vi "E4440A_PSA_Configure_Marker.vi"(0 "VISA resource name":refnum<visa-resource-name>, 1 "X (0 Hz)":dbl, 2 "Center X (0)":dbl, 3 "X Span (0)":dbl, 5 "Active Marker (1: Marker1)":u16(ring)=1 items=["Marker1"=1, "Marker2"=2, "Marker3"=3, "Marker4"=4], 7 "Marker Type (1: Position)":u16(ring)=1 items=["Off", "Position", "Delta", "Band", "Span Pair"], 9 "Readout (0: Frequency)":u16(ring) items=["Frequency", "Time", "Inverse Time", "Period"], 11 "error in (no error)":errorcluster, 12 "X Start (0)":dbl, 13 "X Stop (0)":dbl) -> (4 "VISA resource name out":refnum<visa-resource-name>, 15 "error out":errorcluster)   [LabVIEW 2015]
doc: "Configures the marker type settings of the selected marker."
panel:
  # "Span Pair"
  # "Band"
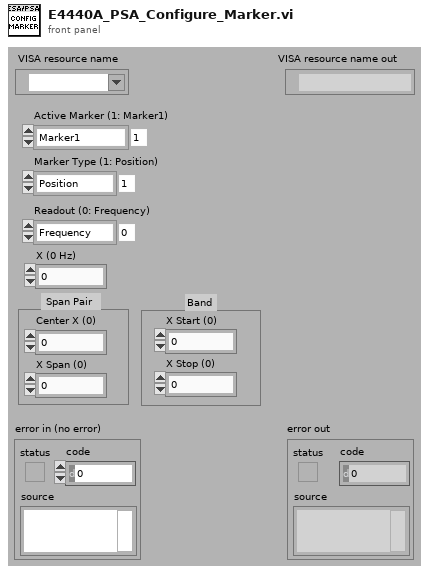
[diagram p1: front panel]
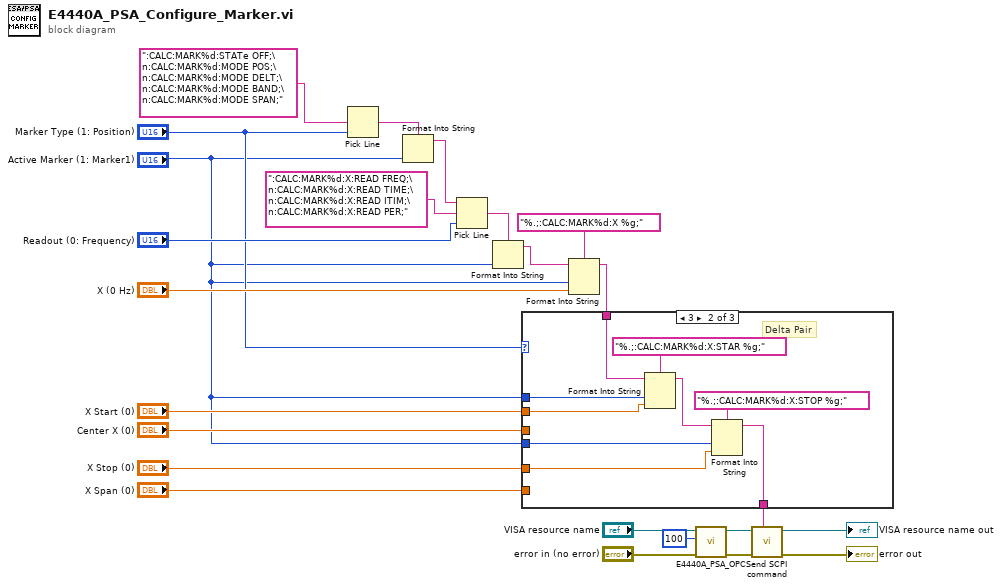
[diagram p0: block diagram]
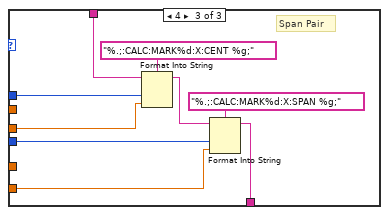
[diagram p3: hidden frame]
diagram:
  n1 = Pick Line(multi-line string=":CALC:MARK%d:STATe OFF;\n:CALC:MARK%d:MODE POS;\n:CALC:MARK%d:MODE DELT;\n:CALC:MARK%d:MODE BAND;\n:CALC:MARK%d:MODE SPAN;", line index="Marker Type (1: Position)") -> (output string=w22:string)  [unwired: 1 in]
  n2 = Format Into String(format string=w22, "Active Marker (1: Marker1)") -> (resulting string=w19:string)  [unwired: 2 in, 1 out]
  n3 = Pick Line(string ("")=w19, multi-line string=":CALC:MARK%d:X:READ FREQ;\n:CALC:MARK%d:X:READ TIME;\n:CALC:MARK%d:X:READ ITIM;\n:CALC:MARK%d:X:READ PER;", line index="Readout (0: Frequency)") -> (output string=w18:string)
  n4 = Format Into String(format string=w18, "Active Marker (1: Marker1)") -> (resulting string=w16:string)  [unwired: 2 in, 1 out]
  n5 = Format Into String(format string="%.;:CALC:MARK%d:X %g;", initial string=w16, "Active Marker (1: Marker1)", "X (0 Hz)") -> (resulting string=w13:string)  [unwired: 1 in, 1 out]
  n6 = case shown="3" "Marker Type (1: Position)" {
    tunnel: "Active Marker (1: Marker1)" -> [_ w31 w39]
    tunnel: "Active Marker (1: Marker1)" -> [_ w30 w38]
    tunnel: w13 -> [w25 w29 w40]
    tunnel: [w25 w28 w37] -> w5
    tunnel: "X Start (0)" -> [_ w27 _]
    tunnel: "X Stop (0)" -> [_ w26 _]
    tunnel: "Center X (0)" -> [_ _ w36]
    tunnel: "X Span (0)" -> [_ _ w35]
    frame 0, Default {
    }
    frame 3 {
      # "Delta Pair"
      n7 = Format Into String(format string="%.;:CALC:MARK%d:X:STAR %g;", initial string=w29, w31, w27) -> (resulting string=w34:string)  [unwired: 1 in, 1 out]
      n8 = Format Into String(format string="%.;:CALC:MARK%d:X:STOP %g;", initial string=w34, w30, w26) -> (resulting string=w28:string)  [unwired: 1 in, 1 out]
    }
    frame 4 {
      # "Span Pair"
      n9 = Format Into String(format string="%.;:CALC:MARK%d:X:CENT %g;", initial string=w40, w39, w36) -> (resulting string=w43:string)  [unwired: 1 in, 1 out]
      n10 = Format Into String(format string="%.;:CALC:MARK%d:X:SPAN %g;", initial string=w43, w38, w35) -> (resulting string=w37:string)  [unwired: 1 in, 1 out]
    }
  }
  n11 = call "E4440A_PSA_OPC.vi"("error in (no error)"="error in (no error)", "Wait (1000ms)"=u32 100, "VISA resource name"="VISA resource name") -> ("error out"=w4:errorcluster, "VISA resource name out"=w2:refnum<visa-resource-name>)  [unwired: 7 in]
  n12 = call "Send SCPI command.vi"("Send SCPI Command"=w5, "error in (no error)"=w4, "VISA resource name"=w2) -> ("error out"=→"error out":errorcluster, "VISA resource name out"=→"VISA resource name out":refnum<visa-resource-name>)  [unwired: 7 in]
